vi "tweak shooter speed.vi"(1 "Increase Z-Axis":dbl=-1.0, 2 "Decrease Z-Axis":dbl=-1.0, 3 "Calculated Speed":dbl) -> (0 "Output Speed":dbl)   [LabVIEW 2011]
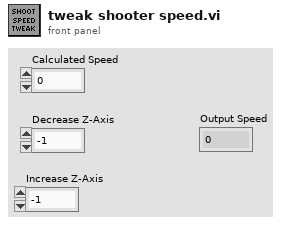
[diagram p1: front panel]
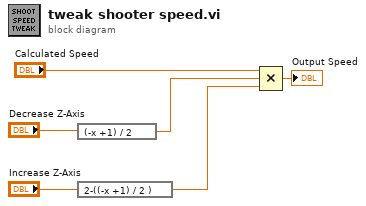
[diagram p0: block diagram]
diagram:
  n1 = expression code="(-x +1) / 2"("Decrease Z-Axis") -> (w3:dbl)
  n2 = expression code="2-((-x +1) / 2 )"("Increase Z-Axis") -> (w2:dbl)
  n3 = Compound Arithmetic op=MULTIPLY("Calculated Speed", w3, w2) -> (→"Output Speed":dbl)
